vi "Am I Turning.vi"(10 "Right Joystick":dbl, 11 "Left Joystick":dbl) -> (3 "Turn?":bool)   [LabVIEW 2013]
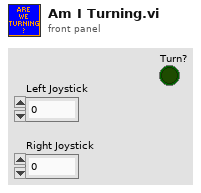
[diagram p1: front panel]
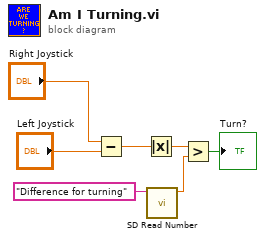
[diagram p0: block diagram]
diagram:
  n1 = Subtract(x="Right Joystick", y="Left Joystick") -> (x-y=w5:dbl)
  n2 = Absolute Value(x=w5) -> (abs(x)=w6:dbl)
  n3 = call <vilib>:"SD Read Number.vi"("Name"="Difference for turning") -> ("Numeric"=w7:dbl)  [unwired: 8 in, 2 out]
  n4 = Greater?(x=w6, y=w7) -> (0:→"Turn?":bool)
